vi "De-Clamp.vi"(7 "Model Name":T1, 8 "Error In":errorcluster, 9 "Intialize?":bool=TRUE, 10 "Inputs":T2) -> (0 "error out":errorcluster, 1 "Completed":bool, 4 "Status":cluster{"Status":string, "Elapsed Time":dbl})   [LabVIEW 2017]
uses:
  controls/All Inputs.ctl
  controls/SACB DI.ctl
  controls/Model Name.ctl
  controls/De-Clamp.ctl
  controls/FGV DO.ctl
panel:
  in  "Delay (for De-Clamp)":u32
  in  "Timeout (ms)":u32=15000
  # "Inputs"
  # "Variables"
  # "Outputs"
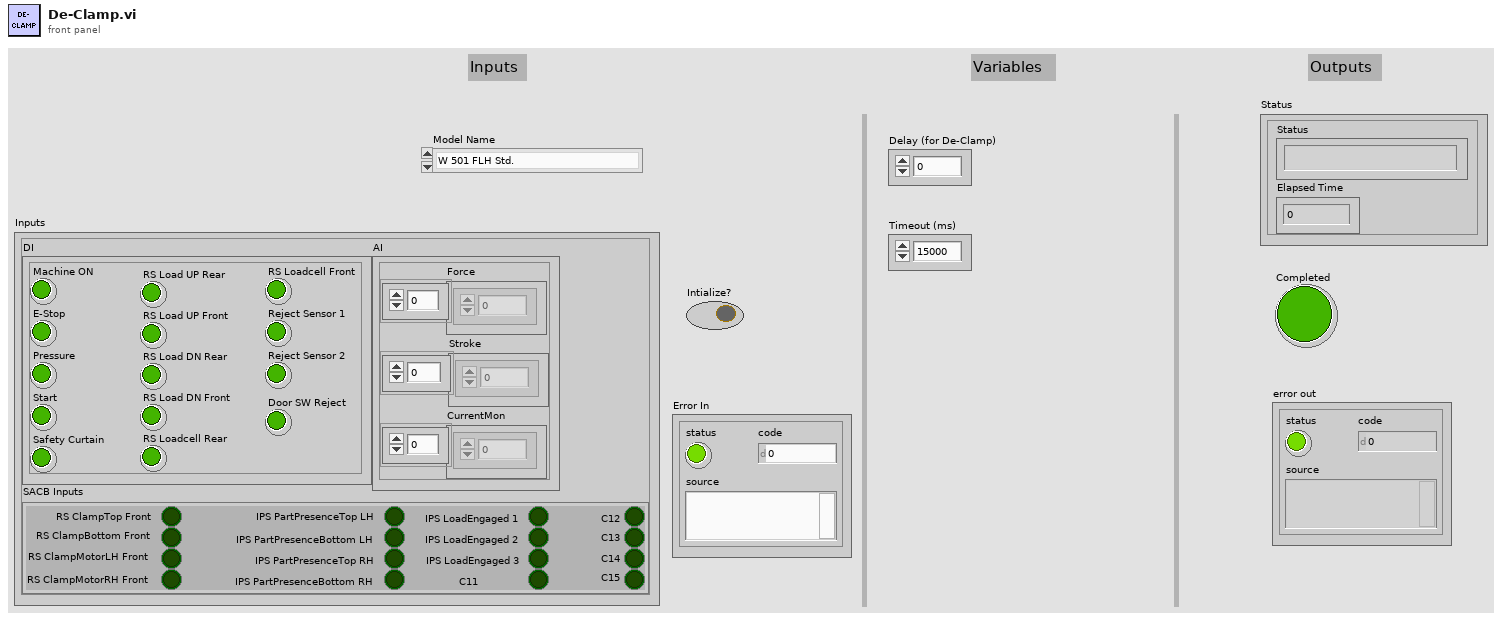
[diagram p1: front panel]
types:
  T1 = typedef "Model Name.ctl" = enum16{"W 501 FLH Std.", "W 501 FRH Std.", "W 601 FR RH Std", "W 601 FR LH Std", "W 601 RR RH Std", "W 601 RR LH Std", "W 601 FR RH AP", "W 601 FR LH AP", "W 601 RR RH AP", "W 601 RR LH AP"}
  T2 = typedef "All Inputs.ctl" = cluster{"DI":cluster{"Machine ON":bool, "E-Stop":bool, "Pressure":bool, "Start":bool, "Safety Curtain":bool, "RS Load UP Rear":bool, "RS Load UP Front":bool, "RS Load DN Rear":bool, "RS Load DN Front":bool, "RS Loadcell Rear":bool, "RS Loadcell Front":bool, "Reject Sensor 1":bool, "Reject Sensor 2":bool, "Door SW Reject":bool}, "AI":cluster{"Force":dbl[], "Stroke":dbl[], "CurrentMon":dbl[]}, "SACB Inputs":T3}
  T3 = typedef "SACB DI.ctl" = cluster{"RS ClampTop Front":bool, "RS ClampBottom Front":bool, "RS ClampMotorLH Front":bool, "RS ClampMotorRH Front":bool, "IPS PartPresenceTop LH":bool, "IPS PartPresenceBottom LH":bool, "IPS PartPresenceTop RH":bool, "IPS PartPresenceBottom RH":bool, "IPS LoadEngaged 1":bool, "IPS LoadEngaged 2":bool, "IPS LoadEngaged 3":bool, "C11":bool, "C12":bool, "C13":bool, "C14":bool, "C15":bool}
  T4 = typedef "De-Clamp.ctl" = enum16{"Initialize", "Disengage Clamping", "Delay (for De-Clamp)", "Done", "Error"}
  T5 = typedef "FGV DO.ctl" = enum16{"Initialize", "Start Task", "Clamping", "Load CYL", "Contactors", "Loadcell CYL", "BSL", "Read DO", "Clear Tasks", "Clear Task"}
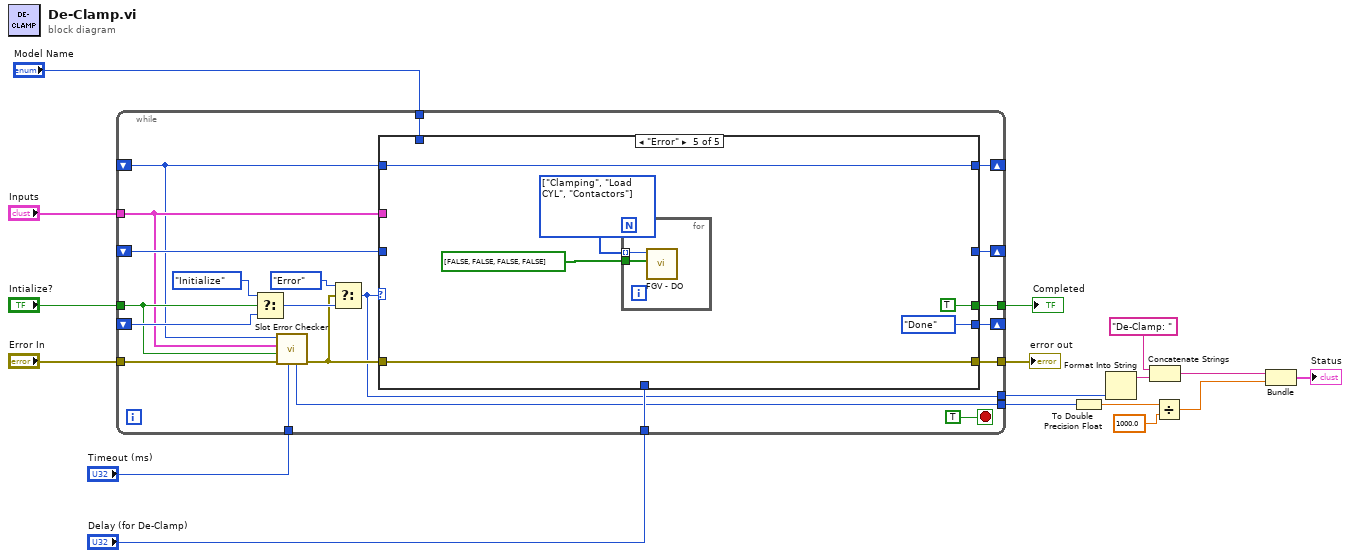
[diagram p0: block diagram]
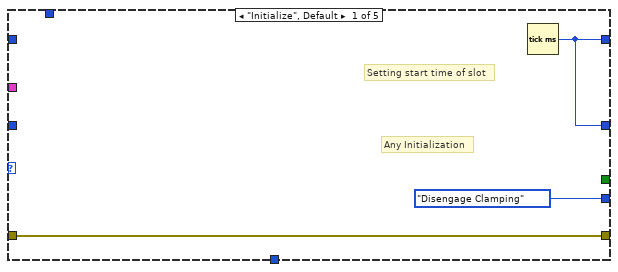
[diagram p2: hidden frame]
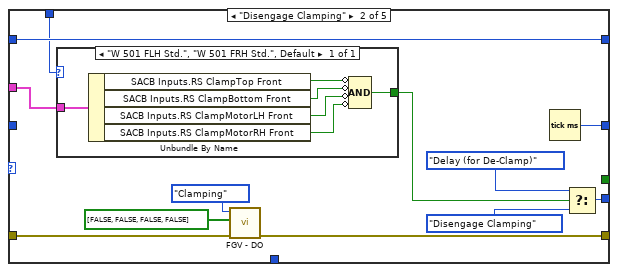
[diagram p3: hidden frame]
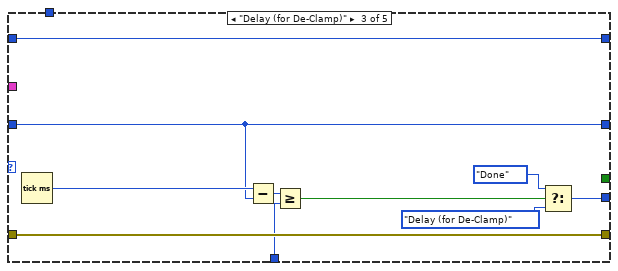
[diagram p4: hidden frame]
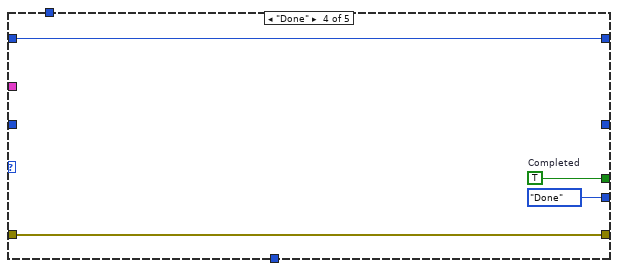
[diagram p5: hidden frame]
diagram:
  n1 = while {
    tunnel: "Intialize?" -> [w28]
    shift-right: [w35] -> _
    shift-left: _ -> [w37]
    shift-right: [w34] -> _
    shift-left: _ -> [w33]
    tunnel: "Error In" -> [w29]
    tunnel: [w32] -> w17
    tunnel: [w31] -> w16
    tunnel: "Inputs" -> [w27]
    shift-right: [w30] -> _
    shift-left: _ -> [w26]
    tunnel: "Delay (for De-Clamp)" -> [w22]
    tunnel: "Timeout (ms)" -> [w21]
    tunnel: [w20] -> w10
    tunnel: [w19] -> w7
    tunnel: "Model Name" -> [w18]
    stop <- TRUE stop-if-true
    n2 = Select(t=De-Clamp."Initialize", s=w28, f=w37) -> (s? t:f=w25:T4)
    n3 = call "Slot Error Checker.vi"("Timeout (ms)"=w21, "error in (no error)"=w29, "Intialize?"=w28, "Inputs"=w27, "start time"=w26) -> ("error out"=w24:errorcluster, "Slot Time"=w19:u32)  [unwired: 5 in]
    n4 = Select(t=De-Clamp."Error", s=w24, f=w25) -> (s? t:f=w20:T4)
    n5 = case shown="\"Error\"" w20 {
      tunnel: [De-Clamp."Disengage Clamping" w45 w66 De-Clamp."Done" De-Clamp."Done"] -> w35
      tunnel: [w39 w49 w68 _ _] -> w34
      tunnel: w33 -> [_ _ w68 _ _]
      tunnel: w24 -> [w40 w53 w64 w72 w79]
      tunnel: [w40 w52 w64 w72 w79] -> w32
      tunnel: [_ _ _ w71 TRUE ("Completed")] -> w31
      tunnel: w27 -> [_ w46 _ _ _]
      tunnel: [w39 w48 w61 w70 w76] -> w30
      tunnel: w26 -> [_ w48 w61 w70 w76]
      tunnel: w22 -> [_ _ w60 _ _]
      tunnel: w18 -> [_ w47 _ _ _]
      frame "Initialize", Default {
        # "Setting start time of slot"
        # "Any Initialization"
        n6 = Tick Count (ms)() -> (millisecond timer value=w39:u32)
      }
      frame "Disengage Clamping" {
        n7 = case shown="\"W 501 FLH Std.\", \"W 501 FRH Std.\", Default" w47 {
          tunnel: w46 -> [w59]
          tunnel: [w54] -> w42
          frame "W 501 FLH Std.", "W 501 FRH Std.", Default {
            n8 = Unbundle By Name(w59) -> ("SACB Inputs.RS ClampTop Front"=w58:bool, "SACB Inputs.RS ClampBottom Front"=w57:bool, "SACB Inputs.RS ClampMotorLH Front"=w56:bool, "SACB Inputs.RS ClampMotorRH Front"=w55:bool)
            n9 = Compound Arithmetic op=AND(invert w58, invert w57, invert w56, invert w55) -> (w54:bool)
          }
        }
        n10 = call "FGV - DO.vi"("error in"=w53, "Digital Outs"=bool[] [FALSE, FALSE, FALSE, FALSE], "State"=FGV_DO."Clamping") -> ("error out"=w52:errorcluster)  [unwired: 7 in, 1 out]
        n11 = Tick Count (ms)() -> (millisecond timer value=w49:u32)
        n12 = Select(t=De-Clamp."Delay (for De-Clamp)", s=w42, f=De-Clamp."Disengage Clamping") -> (s? t:f=w45:T4)
      }
      frame "Delay (for De-Clamp)" {
        n13 = Tick Count (ms)() -> (millisecond timer value=w69:u32)
        n14 = Subtract(x=w69, y=w68) -> (x-y=w67:u32)
        n15 = Greater Or Equal?(x=w67, y=w60) -> (x >= y?=w65:bool)
        n16 = Select(t=De-Clamp."Done", s=w65, f=De-Clamp."Delay (for De-Clamp)") -> (s? t:f=w66:T4)
      }
      frame "Done" {
        w71 = TRUE  # Completed
      }
      frame "Error" {
        w74 = T5[] [enum."Clamping", enum."Load CYL", enum."Contactors"] items=["Initialize", "Start Task", "Clamping", "Load CYL", "Contactors", "Loadcell CYL", "BSL", "Read DO", "Clear Tasks", "Clear Task"]
        n17 = for {
          tunnel: w74 -> [w81] mode=indexing
          tunnel: bool[] [FALSE, FALSE, FALSE, FALSE] ("Digital Outs") -> [w80]
          n18 = call "FGV - DO.vi"("Digital Outs"=w80, "State"=w81) -> ()  [unwired: 8 in, 2 out]
        }
      }
    }
  }
  "error out" <- w17
  "Completed" <- w16
  n19 = To Double Precision Float(number=w7) -> (double precision float=w6:dbl)
  n20 = Format Into String(w10) -> (resulting string=w9:string)  [unwired: 3 in, 1 out]
  n21 = Concatenate Strings("De-Clamp: ", w9) -> (w4:string)
  n22 = Divide(x=w6, y=1000.0) -> (x/y=w3:dbl)
  n23 = Bundle(w4, w3) -> (→"Status":cluster{string, dbl})  [unwired: 1 in]
